vi "Constructor.vi"(8 "error in (no error)":errorcluster, 11 "VIActivation in":refnum<class "VIActivation.lvclass">) -> (0 "error out":errorcluster, 2 "VIActivation":refnum<event-registration>, 3 "VIActivation out":refnum<class "VIActivation.lvclass">)   [LabVIEW 2021, in "VIActivation.lvlib" / "VIActivation.lvclass"]
uses:
  VIActivation.lvclass
  VIActivationEvents.ctl
  GetVIActivationEvent.vi
  GetVIDesactivationEvent.vi
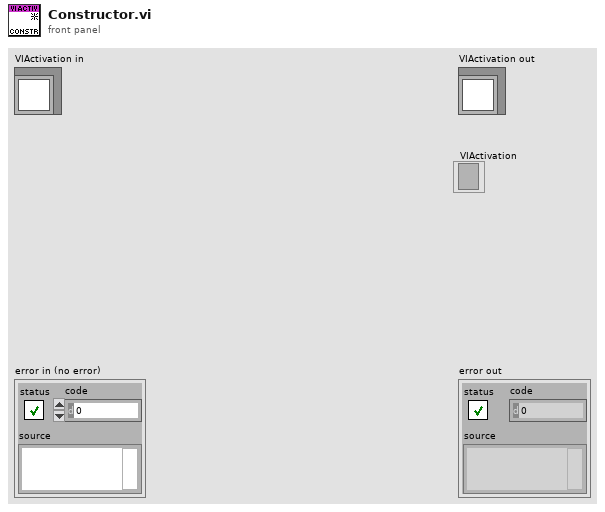
[diagram p1: front panel]
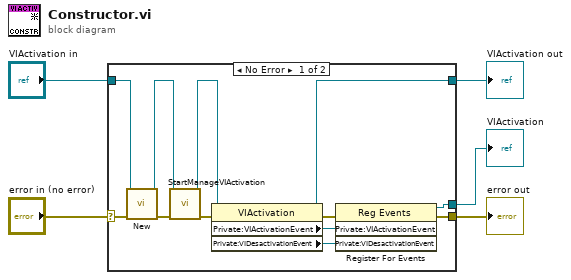
[diagram p0: block diagram]
diagram:
  n1 = case shown="No Error" "error in (no error)" {
    selector: "error in (no error)" -> [w7 w19]
    tunnel: [w15 w19] -> w4
    tunnel: [w11 w18] -> w2
    tunnel: "VIActivation in" -> [w10 w18]
    tunnel: [w12 _] -> w1
    frame No Error {
      n2 = call-dynamic "New.vi"("error in (no error)"=w7, "ByRefClass in"=w10) -> ("error out"=w8:errorcluster, "ByRefClass out"=w9:refnum<class "VIActivation.lvclass">)  [unwired: 8 in]
      n3 = call "StartManageVIActivation.vi"("error in (no error)"=w8, "Menu in"=w9) -> ("error out"=w6:errorcluster, "Menu out"=w16:refnum<class "VIActivation.lvclass">)  [unwired: 8 in]
      n4 = property class="VIActivation"(reference=w16, error in=w6) -> (reference out=w11:refnum<class "VIActivation.lvclass">, error out=w17:errorcluster, "Private:VIActivationEvent"=w14:refnum<user-event>, "Private:VIDesactivationEvent"=w13:refnum<user-event>)
      n5 = register-events(error in=w17, w14, w13) -> (reference out=w12:refnum<event-registration>, error out=w15:errorcluster)  [unwired: 1 in]
    }
    frame Error {
    }
  }
  "error out" <- w4
  "VIActivation out" <- w2
  "VIActivation" <- w1
